vi "send_image.vi"(8 "error in (no error)":errorcluster, 10 "img in":T1, 11 "WebSocket in":refnum<class "WebSocket.lvclass">) -> (0 "error out":errorcluster, 3 "WebSocket out":refnum<class "WebSocket.lvclass">)   [LabVIEW 2018]
uses:
  <vilib>/MediaMongrels Ltd/WebSockets/WebSockets/WebSocket/WebSocket.lvclass
  <vilib>/vision/Image Controls.llb/IMAQ Image.ctl
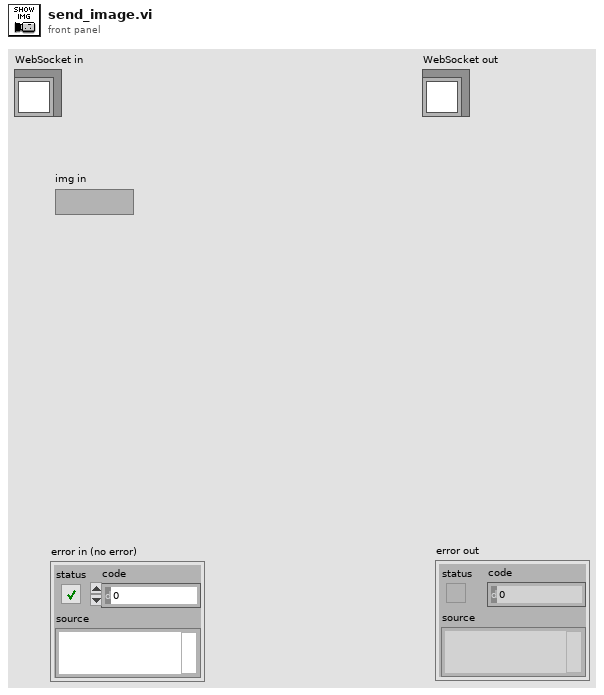
[diagram p1: front panel]
types:
  T1 = typedef "IMAQ Image.ctl" = refnum<image>
  T2 = cluster{"cmd":string, "data":string, "dtype":string}
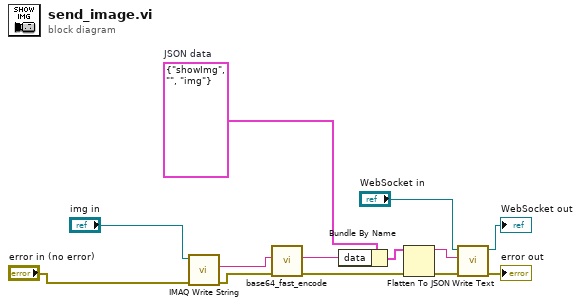
[diagram p0: block diagram]
diagram:
  w8 = T2 {"cmd"="showImg", "data"="", "dtype"="img"}  # JSON data
  n1 = call-poly "IMAQ Write String"("error in (no error)"="error in (no error)", "Image"="img in") -> ("error out"=w2:errorcluster, "FileString"=w1:string)  [unwired: 7 in, 1 out]
  n2 = call "base64_fast_encode.vi"("error in (no error)"=w2, "string in (not encoded)"=w1) -> ("error out"=w5:errorcluster, "string out (base64-encoded)"=w6:string)  [unwired: 8 in]
  n3 = Bundle By Name(cluster=w8, "data"=w6) -> (w7:T2)
  n4 = Flatten To JSON(anything=w7, error in (no error)=w5) -> (JSON string=w12:string, 11:w13:errorcluster)  [unwired: 1 in]
  n5 = call-dynamic "Write Text.vi"("error in (no error)"=w13, "String Data"=w12, "WebSocket in"="WebSocket in") -> ("error out"=→"error out":errorcluster, "WebSocket out"=→"WebSocket out":refnum<class "WebSocket.lvclass">)  [unwired: 7 in]
